vi "Test_StructureSubdiagramsAndDeleteObject.vi"() -> ()   [LabVIEW 2025]
uses:
  8cebb4ce-4f0f-4319-9f7e-82e401bee674.vi
  ff6ee880-e87d-4ac2-b0b9-a7c0f406254d.vi
  57ba1f44-eecb-4af5-975d-0cda700306c1.vi
  Scripting Server.lvlib
panel:
  out "help_string":string
  out "result":string
  out "error out":errorcluster
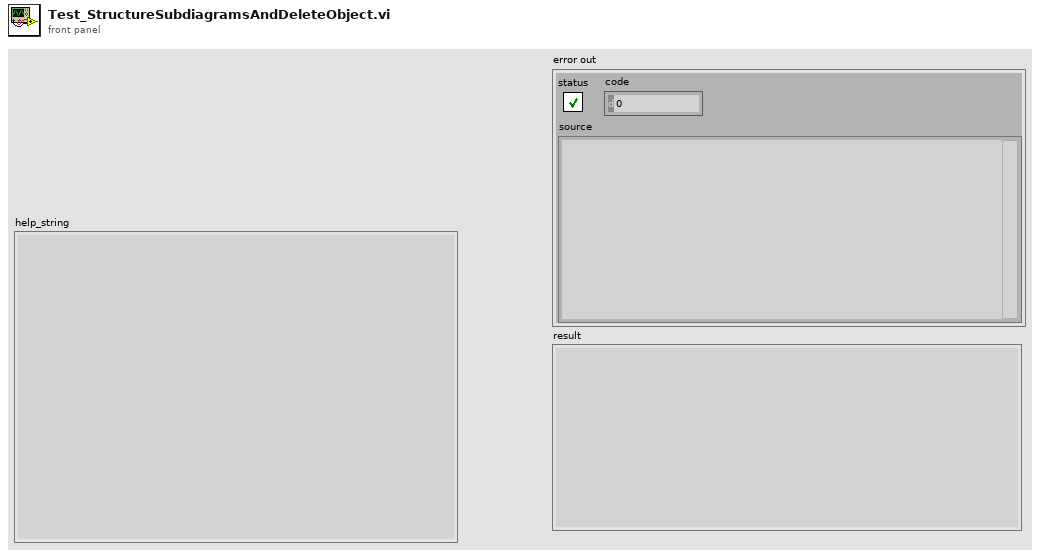
[diagram p1: front panel]
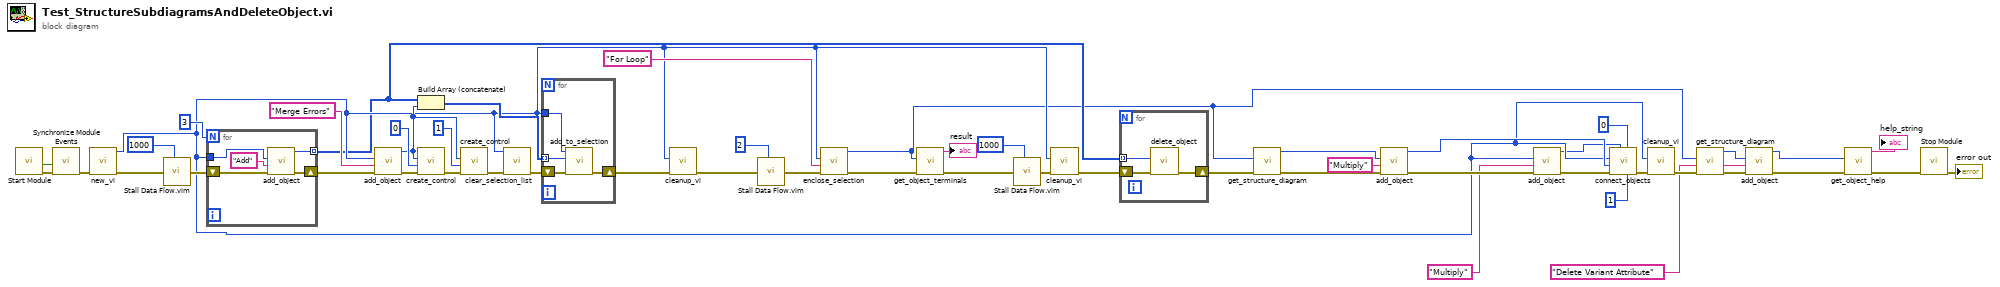
[diagram p0: block diagram]
diagram:
  n1 = call "Start Module.vi"() -> ("error out"=w51:errorcluster, "Wait for Event Sync?"=w52:bool)  [unwired: 7 in, 3 out]
  n2 = call "Synchronize Module Events.vi"("error in"=w51, "Wait for Event Sync?"=w52) -> ("error out"=w50:errorcluster)  [unwired: 9 in]
  n3 = call "new_vi.vi"("error in"=w50) -> ("error out"=w49:errorcluster, "vi_id"=w11:i32)  [unwired: 7 in, 2 out]
  n4 = call "Stall Data Flow.vim"("value in"=w49, "milliseconds to wait"=u32 1000) -> ("value out"=w48:errorcluster)  [unwired: 1 out]
  n5 = for {
    N: 3 -> [_]
    shift-right: [w56] -> w46
    shift-left: w48 -> [w57]
    tunnel: w11 -> [w53]
    tunnel: [w55] -> w10 mode=indexing
    n6 = call "add_object.vi"("error in"=w57, "object_name"="Add", "diagram_id"=w53) -> ("error out"=w56:errorcluster, "object_id"=w55:i32)  [unwired: 5 in, 2 out]
  }
  n7 = call "add_object.vi"("error in"=w46, "object_name"="Merge Errors", "diagram_id"=w11) -> ("error out"=w41:errorcluster, "object_id"=w33:i32)  [unwired: 5 in, 2 out]
  n8 = Build Array (concatenate)(w10, w33) -> (w23:i32[])
  n9 = call "create_control.vi"("error in"=w41, "terminal_index"=0, "object_id"=w33) -> ("error out"=w39:errorcluster)  [unwired: 6 in, 2 out]
  n10 = call "create_control.vi"("error in"=w39, "terminal_index"=1, "object_id"=w33) -> ("error out"=w37:errorcluster)  [unwired: 6 in, 2 out]
  n11 = call "clear_selection_list.vi"("error in"=w37, "vi_id"=w11) -> ("error out"=w35:errorcluster)  [unwired: 8 in, 1 out]
  n12 = for {
    tunnel: w11 -> [w59]
    tunnel: w23 -> [w58] mode=indexing
    shift-right: [w60] -> w34
    shift-left: w35 -> [w61]
    n13 = call "add_to_selection.vi"("error in"=w61, "object_id"=w58, "vi_id"=w59) -> ("error out"=w60:errorcluster)  [unwired: 7 in, 1 out]
  }
  n14 = call "cleanup_vi.vi"("error in"=w34, "vi_reference"=w11) -> ("error out"=w27:errorcluster)  [unwired: 7 in, 2 out]
  n15 = call "Stall Data Flow.vim"("value in"=w27, "milliseconds to wait"=u32 2) -> ("value out"=w30:errorcluster)  [unwired: 1 out]
  n16 = call "enclose_selection.vi"("error in"=w30, "structure_type"="For Loop", "vi_id"=w11) -> ("error out"=w32:errorcluster, "object_id"=w2:i32)  [unwired: 6 in, 1 out]
  n17 = call "get_object_terminals.vi"("error in"=w32, "object_id"=w2) -> ("error out"=w26:errorcluster, "result"=→"result":string)  [unwired: 7 in, 1 out]
  n18 = call "Stall Data Flow.vim"("value in"=w26, "milliseconds to wait"=u32 1000) -> ("value out"=w45:errorcluster)  [unwired: 1 out]
  n19 = call "cleanup_vi.vi"("error in"=w45, "vi_reference"=w11) -> ("error out"=w43:errorcluster)  [unwired: 7 in, 2 out]
  n20 = for {
    tunnel: w10 -> [w62] mode=indexing
    shift-right: [w63] -> w24
    shift-left: w43 -> [w64]
    n21 = call "delete_object.vi"("error in"=w64, "object_id"=w62) -> ("error out"=w63:errorcluster)  [unwired: 8 in, 1 out]
  }
  n22 = call "get_structure_diagram.vi"("error in"=w24, "structure_id"=w2) -> ("error out"=w22:errorcluster, "diagram_id"=w20:i32)  [unwired: 7 in, 1 out]
  n23 = call "add_object.vi"("error in"=w22, "object_name"="Multiply", "diagram_id"=w20) -> ("error out"=w21:errorcluster, "object_id"=w15:i32)  [unwired: 5 in, 2 out]
  n24 = call "add_object.vi"("error in"=w21, "object_name"="Multiply", "diagram_id"=w11) -> ("error out"=w18:errorcluster, "object_id"=w7:i32)  [unwired: 5 in, 2 out]
  n25 = call "connect_objects.vi"("to_object_terminal_index"=1 ("from_object_terminal_index"), "from_object_terminal_index"=0, "to_object_reference"=w7, "error in"=w18, "from_object_reference"=w15, "vi_reference"=w11) -> ("error out"=w16:errorcluster)  [unwired: 3 in, 2 out]
  n26 = call "cleanup_vi.vi"("error in"=w16, "vi_reference"=w11) -> ("error out"=w12:errorcluster)  [unwired: 7 in, 2 out]
  n27 = call "get_structure_diagram.vi"("error in"=w12, "structure_id"=w2) -> ("error out"=w3:errorcluster, "diagram_id"=w1:i32)  [unwired: 7 in, 1 out]
  n28 = call "add_object.vi"("error in"=w3, "object_name"="Delete Variant Attribute", "diagram_id"=w1) -> ("error out"=w6:errorcluster, "object_id"=w4:i32)  [unwired: 5 in, 2 out]
  n29 = call "get_object_help.vi"("error in"=w6, "object_id"=w4) -> ("error out"=w9:errorcluster, "help_string"=→"help_string":string)  [unwired: 7 in, 1 out]
  n30 = call "Stop Module.vi"("error in"=w9) -> ("error out"=→"error out":errorcluster)  [unwired: 10 in]
